vi "CRYASIOOpenOutputWave.vi"(5 "Buff Length":u32=100, 6 "Channel Index":u32, 7 "Buff Count":u32=20, 8 "Bit Depth":u16=16, 9 "Sampling Rate":u32=44100, 10 "error in (no error)":errorcluster) -> (1 "OCI":u32, 2 "bResult":bool, 3 "error out":errorcluster)   [LabVIEW 2013]
uses:
  CRY_ASIO.dll
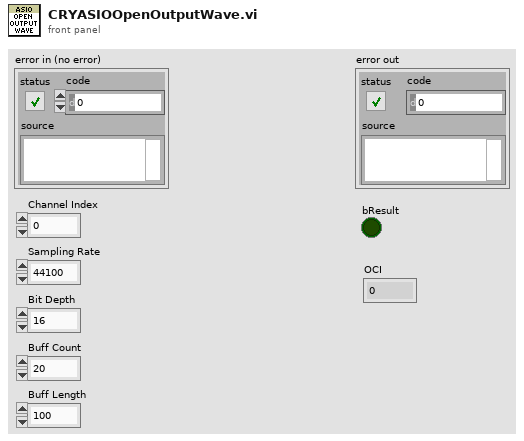
[diagram p1: front panel]
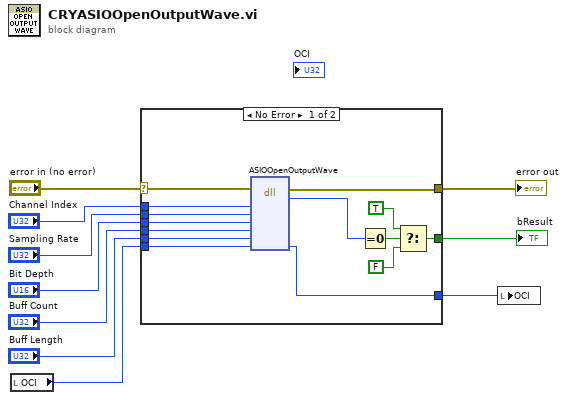
[diagram p0: block diagram]
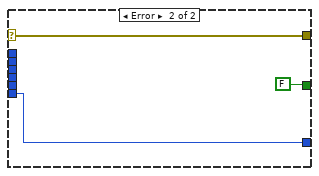
[diagram p2: hidden frame]
diagram:
  n1 = local read "OCI"() -> (w2:u32)
  n2 = case shown="No Error" "error in (no error)" {
    selector: "error in (no error)" -> [w20 w27]
    tunnel: [w19 w27] -> w9
    tunnel: [w21 FALSE] -> w8
    tunnel: "Channel Index" -> [w17 _]
    tunnel: "Sampling Rate" -> [w16 _]
    tunnel: "Bit Depth" -> [w15 _]
    tunnel: "Buff Count" -> [w14 _]
    tunnel: "Buff Length" -> [w13 _]
    tunnel: w2 -> [w12 w25]
    tunnel: [w11 w25] -> w1
    frame No Error {
      n3 = dll-call lib="D:/LabView_Project/CRY6181/CRY_ASIO.dll" fn="ASIOOpenOutputWave"(error in=w20, "arg1"=w17, "arg2"=w16, "arg3"=w15, "arg4"=w14, "arg5"=w13, "arg6"=w12) -> (error out=w19:errorcluster, "return type"=w18:u32, "arg6"=w11:u32)  [unwired: 7 in, 1 out]
      n4 = Equal To 0?(x=w18) -> (x = 0?=w24:bool)
      n5 = Select(t=TRUE, s=w24, f=FALSE) -> (s? t:f=w21:bool)
    }
    frame Error {
    }
  }
  "error out" <- w9
  "bResult" <- w8
  n6 = local write "OCI"(w1) -> ()
